vi "FXP_LinearControlLaw_singleAxis_uk_and_deltauk.vi"(7 "ControlParams_distEst":T1={"umax"=3.0, "NS"=0, "ref_f_VEC"=[0.0, 0.0], "Nu11_22"=[0.0, 0.0], "u0"=[0.0, 0.0]} {"ref_f_VEC" format="%#_9g"}, 8 "yd_est_x":fxp<+/-,32,5>, 9 "du_max":fxp<+/-,18,5>) -> (0 "del u_x":fxp<+/-,64,15>, 2 "u_k (saturated)":fxp<+/-,32,5>, 3 "saturated?":bool, 6 "xerr":fxp<+/-,32,5>[](array[numeric]))   [LabVIEW 2017]
uses:
  typeDefs/FXPControlParams_distEst.ctl
  <vilib>/Platform/TimedLoop/XDataNode/timing_clust.ctl
  <vilib>/Platform/TimedLoop/XDataNode/nitl_modes.ctl
  <vilib>/Platform/TimedLoop/XDataNode/wakeup.ctl
  typeDefs/x_vec_bram.ctl
  <vilib>/rvi/Emulation/niFpgaSctlEmulationGetInTimedLoop.vi
  <vilib>/rvi/Emulation/niFpgaEmulationReportErrorSimple.vi
  <vilib>/rvi/Emulation/niFpgaGetClockAttributes.vi
  <vilib>/rvi/Emulation/niFpgaCriticalErrorInLSC.vi
  <vilib>/rvi/DataTransferAndStorage/Container/Common/niFpgaContainerExecOnDevCompGetState.vi
  <vilib>/rvi/Emulation/niFpgaEmulationIsFPGAContextNoSignature.vi
  <vilib>/rvi/DataTransferAndStorage/Container/Common/niFpgaContainerGetUniqueNameForEmu.vi
  <vilib>/rvi/Emulation/niFpgaProcessEmulError.vi
  <vilib>/rvi/errors/nirviReportUnexpectedCaseInternalError (U32).vi
  <vilib>/rvi/Memory/Memory_Emulation/niFpgaMemoryEmulationCacheClearOnFirstRun.vi
  <vilib>/rvi/Memory/Memory_Emulation/nirvimemoryEmulationManagerCache_MakeExclusive.vi
  <vilib>/rvi/Memory/Memory_Emulation/niFpgaMemoryEmulationValidateCache.vi
  <vilib>/rvi/Memory/Memory_Emulation/nirvimemoryEmulationManagerCache_InsertValue.vi
  <vilib>/Utility/error.llb/Clear Errors.vi
  <vilib>/rvi/Memory/Memory_Emulation/nirvimemoryEmulationManagerCache_ReleaseExclusive.vi
  <vilib>/rvi/Memory/Memory_Emulation/nirvimemoryEmulationManagerCache_GetValue.vi
  <vilib>/rvi/Memory/Memory_Emulation/nirvimemoryEmulationManagerCache_SetValue.vi
  <vilib>/rvi/Emulation/niFpgaSctlEmulationResourceMgr.vi
  <vilib>/Platform/TimedLoop/XDataNode/XDataNode.xnode
  <vilib>/rvi/FXPMathLib/FxpAdd/XNode/nifxpmath_Add.xnode
  <vilib>/rvi/DataTransferAndStorage/Container/XNode/niFpgaContainer.xnode
  <vilib>/rvi/Memory/Memory_Emulation/niFpgaMemoryEmulationRefIn.vi
  <vilib>/Platform/TimedLoop/XDataNode/XDNodeRunTimeDep.lvlib
  <vilib>/rvi/FXPMathLib/sim/FxpSim.dll
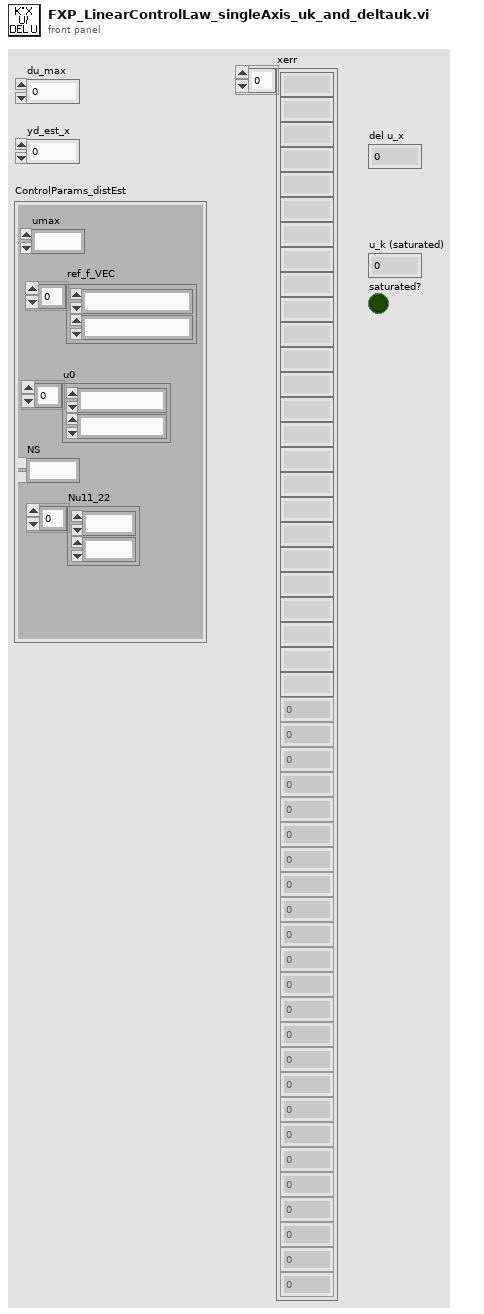
[diagram p1: front panel]
types:
  T1 = typedef "FXPControlParams_distEst.ctl" = cluster{"umax":fxp<+/-,18,5>, "NS":u8, "ref_f_VEC":fxp<+/-,32,5>[], "Nu11_22":fxp<+/-,32,5>[], "u0":fxp<+/-,32,5>[]}
  T2 = typedef "x_control.ctl" = fxp<+/-,18,5>[]
  T3 = typedef "XDNodeRunTimeDep.lvlib/timing_clust.ctl" = cluster{"Expected End [f-1]":u64, "Actual End [f-1]":u64, "Finished Late? [f-1]":bool, "Expected End [i-1]":u64, "Actual End [i-1]":u64, "Finished Late? [i-1]":bool, "Expected Start [i]":u64, "Actual Start [i]":u64, "Expected Start [f]":u64, "Actual Start [f]":u64, "Source Name":string, "Structure Name":string, "Period":i64, "Deadline":i64, "Offset":i64, "Start":i64, "Priority":i32, "Timeout":i32, "Mode":T4, "Wakeup Reason":T5, "Error":errorcluster, "Source Type":string, "Secondary Source Type":string, "Global End Time":u64, "Global Start Time":u64, "Frame Duration":u64, "Iteration Duration":u64, "Assigned CPU":i32, "I/O Scan Engine Mode":u32}
  T4 = typedef "XDNodeRunTimeDep.lvlib/nitl_modes.ctl" = enum32{"No Change", "Process missed periods, maintain original phase", "Discard missed periods, maintain original phase", "Process missed periods, ignore original phase", "Discard missed periods, ignore original phase"}
  T5 = typedef "XDNodeRunTimeDep.lvlib/wakeup.ctl" = enum32{"Normal", "Aborted", "Asynchronous wakeup", "Timing source error", "Timed loop error", "Timeout"}
  T6 = typedef "x_vec_bram.ctl" = refnum<k21>
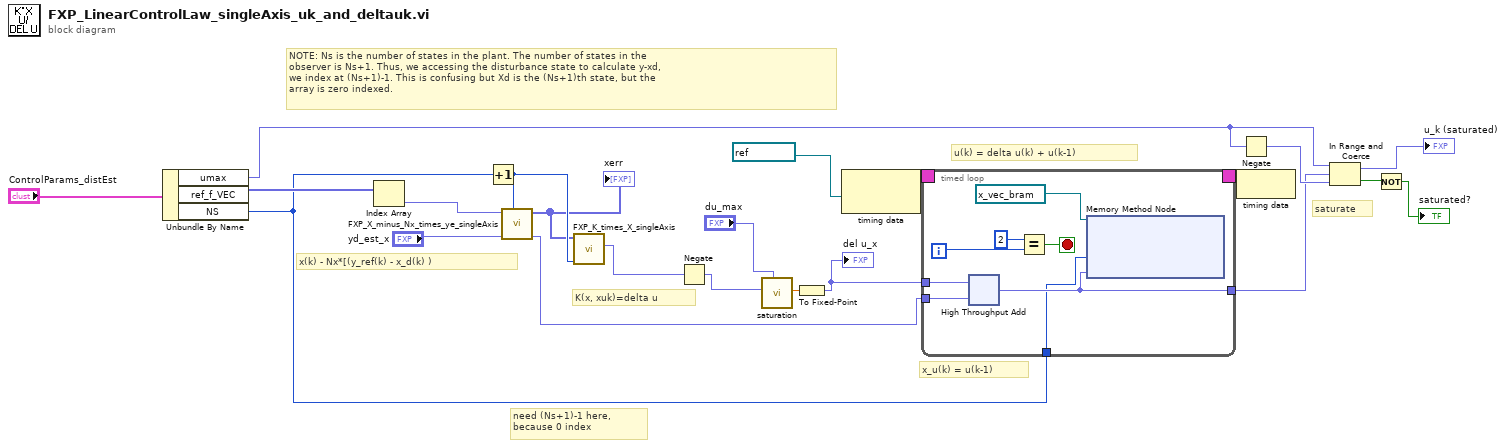
[diagram p0: block diagram]
diagram:
  # "saturate"
  # "need (Ns+1)-1 here,\nbecause 0 index"
  # "K(x, xuk)=delta u"
  # "u(k) = delta u(k) + u(k-1)"
  # "x_u(k) = u(k-1)"
  # "x(k) - Nx*[(y_ref(k) - x_d(k) )"
  # "NOTE: Ns is the number of states in the plant. The number of states in the \nobserver is Ns+1. Thus, we accessing the disturbance state to calculate y-xd, \nwe index at (Ns+1)-1. This is confusing but Xd is the (Ns+1)th state, but the \narray is zero indexed."
  n1 = Unbundle By Name("ControlParams_distEst") -> ("umax"=w3:fxp<+/-,18,5>, "ref_f_VEC"=w18:fxp<+/-,32,5>[], "NS"=w7:u8)
  n2 = Index Array(array=w18) -> (element=w19:fxp<+/-,32,5>)  [unwired: 1 in]
  n3 = Increment(x=w7) -> (x+1=w10:u8)
  n4 = call "FXP_X_minus_Nx_times_ye_singleAxis.vi"("NS"=w10, "yd_est_x"="yd_est_x", "ref(k)_x"=w19) -> ("xu_k"=w8:fxp<+/-,32,5>, "xerr"=w9:T2)  [unwired: 7 in]
  "xerr" <- w9
  n5 = call "FXP_K_times_X_singleAxis.vi"("NS + 1"=w10, "x_vec"=w9) -> ("del u_x"=w12:fxp<+/-,64,15>)  [unwired: 9 in]
  n6 = Negate(x=w12) -> (-x=w11:fxp<+/-,64,16>)
  n7 = call "saturation.vi"("uMax"="du_max", "signal in"=w11) -> ("signal out"=w13:sgl)  [unwired: 8 in, 1 out]
  n8 = To Fixed-Point(number=w13) -> (fixed-point=w17:fxp<+/-,32,6>)  [unwired: 1 in]
  "del u_x" <- w17
  n9 = node-c288(refnum<k21> "80MHz" ("Source Name")) -> (w16:T3)
  n10 = timed-loop {
    timing: w16 -> [_]
    timing-out: [_] -> w15
    tunnel: [w25] -> w1
    tunnel: w8 -> [w30]
    tunnel: w17 -> [w26]
    tunnel: w7 -> [w24]
    i -> [w28]
    stop <- w29 stop-if-true
    n11 = xnode ("High Throughput Add")("x"=w26, "y"=w30) -> ("x+y"=w25:fxp<+/-,32,5>)
    n12 = Equal?(x=2, y=w28) -> (x = y?=w29:bool)
    n13 = xnode ("Memory Method Node")("Address"=w24, "Data"=w25, "Memory In"=T6 "xk_1_2" ("Memory")) -> ()  [unwired: 1 out]
  }
  n14 = node-c288(w15) -> ()
  n15 = Negate(x=w3) -> (-x=w2:fxp<+/-,18,5>)
  n16 = In Range and Coerce(upper limit=w3, x=w1, lower limit=w2) -> (coerced(x)=→"u_k (saturated)":fxp<+/-,32,5>, In Range?=w5:bool)
  n17 = Not(x=w5) -> (.not. x?=→"saturated?":bool)
